vi "GEA2 Read ERD Multiple Messages.vi"(0 "GEA2 Reference In":refnum<k24>, 1 "Retry Count":i32=2 min=0 max=255 step=1, 2 "Read Timeout (ms)":u32=500, 5 "GEA Inputs":T4 {"Destination" format="%.0x"; "Source" format="%.0x"}, 7 "Read ERD List":T2[](array[typedef]) {"ERD Number" format="%.0x"}, 11 "Error In":errorcluster, 12 "#ERDs per message":i32=1 min=1 step=1, 13 "Verify ERD Response?":bool=TRUE, 14 "Low Level Retry Count":u8=3 min=1 step=1) -> (4 "GEA2 Reference Out":refnum<k24>, 6 "Raw Data Out":string[](array[string]), 8 "ERD Data Out":T1[](array[typedef]) {"ERD Number" format="%.0x"}, 15 "Error Out":errorcluster)   [LabVIEW 2016, in "GEA2_Toolkit.lvlib"]
uses:
  library/GEA2_Toolkit.lvlib
  C:/Users/220038920/Desktop/GEA3 Toolkit/GEA3 DLL Source/GeaCommunication.dll
  GEA3 DLL Source/GeaCommunication.dll
  type defs/Source_Destination.ctl
  type defs/ERD Read Data In.ctl
  type defs/Data Type.ctl
  type defs/ERD Read Data Out.ctl
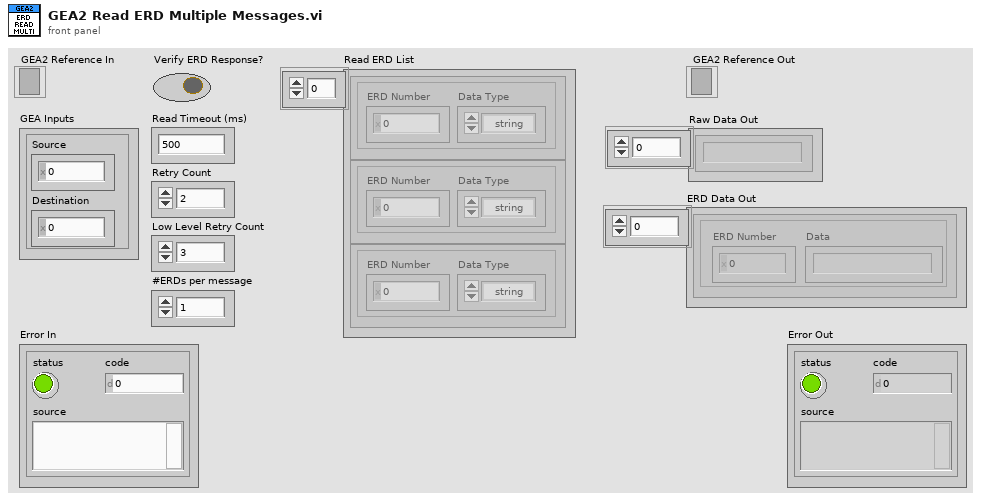
[diagram p1: front panel]
types:
  T1 = typedef "GEA2_Toolkit.lvlib/ERD Read Data Out.ctl" = cluster{"ERD Number":u16, "Data":string}
  T2 = typedef "GEA2_Toolkit.lvlib/ERD Read Data In.ctl" = cluster{"ERD Number":u16, "Data Type":T3}
  T3 = typedef "GEA2_Toolkit.lvlib/Data Type.ctl" = enum16{"string", "boolean", "uint8_t", "uint16_t", "uint32_t", "uint64_t", "int8_t", "int16_t", "int32_t", "int64_t"}
  T4 = typedef "GEA2_Toolkit.lvlib/Source_Destination.ctl" = cluster{"Source":u8, "Destination":u8}
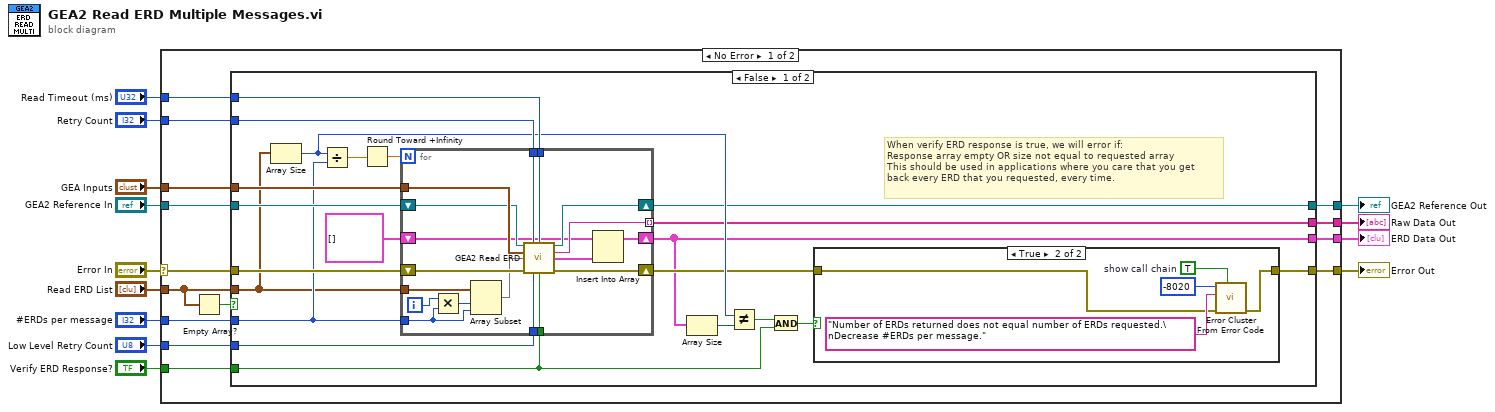
[diagram p0: block diagram]
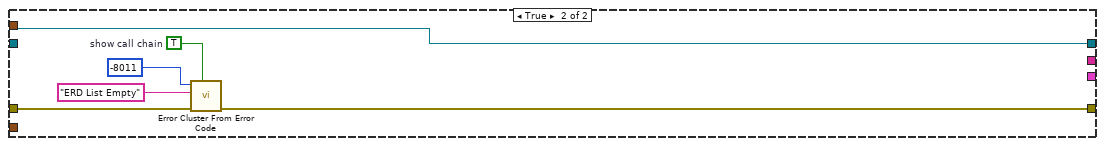
[diagram p3: hidden frame]
diagram:
  n1 = case shown="No Error" "Error In" {
    selector: "Error In" -> [w14 w79]
    tunnel: [w27 w80] -> w13
    tunnel: [w26 w79] -> w12
    tunnel: "Verify ERD Response?" -> [w25 _]
    tunnel: "GEA Inputs" -> [w24 _]
    tunnel: "Read Timeout (ms)" -> [w23 _]
    tunnel: "Retry Count" -> [w22 _]
    tunnel: "GEA2 Reference In" -> [w21 w80]
    tunnel: "#ERDs per message" -> [w20 _]
    tunnel: [w19 _] -> w5
    tunnel: [w18 _] -> w4
    tunnel: "Read ERD List" -> [w17 _]
    tunnel: "Low Level Retry Count" -> [w15 _]
    frame No Error {
      n2 = Empty Array?(array=w17) -> (empty?=w16:bool)
      n3 = case shown="False" w16 {
        tunnel: [w31 w73] -> w27
        tunnel: w14 -> [w48 w75]
        tunnel: [w34 w74] -> w26
        tunnel: w25 -> [w30 _]
        tunnel: w24 -> [w47 _]
        tunnel: w23 -> [w46 _]
        tunnel: w22 -> [w45 _]
        tunnel: w21 -> [w44 w73]
        tunnel: w20 -> [w41 _]
        tunnel: [w32 _] -> w19
        tunnel: [w33 _] -> w18
        tunnel: w17 -> [w38 _]
        tunnel: w15 -> [w39 _]
        frame False {
          # "When verify ERD response is true, we will error if:\nResponse array empty OR size not equal to requested array\nThis should be used in applications where you care that you get\nback every ERD that you requested, every time."
          n4 = Array Size(array=w38) -> (size(s)=w37:i32)
          n5 = Divide(x=w37, y=w41) -> (x/y=w43:dbl)
          n6 = Round Toward +Infinity(x=w43) -> (ceil(x): smallest int >= x=w42:dbl)
          n7 = for {
            N: w42 -> [_]
            tunnel: w30 -> [w69]
            tunnel: w47 -> [w68]
            tunnel: [w67] -> w32 mode=indexing
            tunnel: w46 -> [w66]
            tunnel: w45 -> [w65]
            shift-right: [w72] -> w31
            shift-left: w44 -> [w60]
            shift-right: [w70] -> w35
            shift-left: w48 -> [w71]
            tunnel: w38 -> [w64]
            tunnel: w41 -> [w63]
            shift-right: [w56] -> w33
            shift-left: T1[] [] -> [w58]
            tunnel: w39 -> [w55]
            i -> [w62]
            n8 = Multiply(x=w62, y=w63) -> (x*y=w61:i32)
            n9 = Array Subset(array=w64, index=w61, length=w63) -> (w59:T2[])
            n10 = call "GEA2 Read ERD.vi"("GEA2 Reference In"=w60, "Retry Count"=w65, "Read Timeout (ms)"=w66, "GEA Inputs"=w68, "Read ERD List"=w59, "Error In"=w71, "Low Level Tries"=w55, "Verify ERD Response?"=w69) -> ("GEA2 Reference Out"=w72:refnum<k24>, "Raw Data Out"=w67:string, "ERD Data Out"=w57:T1[], "Error Out"=w70:errorcluster)  [unwired: 4 in]
            n11 = Insert Into Array(array=w58, new element=w57) -> (w56:T1[])  [unwired: 1 in]
          }
          n12 = Array Size(array=w33) -> (size(s)=w36:i32)
          n13 = Not Equal?(x=w37, y=w36) -> (x != y?=w28:bool)
          n14 = And(x=w28, y=w30) -> (x .and. y?=w29:bool)
          n15 = case shown="True" w29 {
            tunnel: w35 -> [w49 w51]
            tunnel: [w49 w50] -> w34
            frame False {
            }
            frame True {
              w54 = TRUE  # show call chain
              n16 = call <vilib>:"Error Cluster From Error Code.vi"("show call chain? (False)"=w54, "error in (no error)"=w51, "error message (\"\")"="Number of ERDs returned does not equal number of ERDs requested.\nDecrease #ERDs per message." ("error message (\"\")"), "error code (0)"=-8020) -> ("error out"=w50:errorcluster)  [unwired: 5 in]
            }
          }
        }
        frame True {
          w76 = TRUE  # show call chain
          n17 = call <vilib>:"Error Cluster From Error Code.vi"("show call chain? (False)"=w76, "error in (no error)"=w75, "error message (\"\")"="ERD List Empty" ("error message (\"\")"), "error code (0)"=-8011) -> ("error out"=w74:errorcluster)  [unwired: 5 in]
        }
      }
    }
    frame Error {
    }
  }
  "GEA2 Reference Out" <- w13
  "Error Out" <- w12
  "Raw Data Out" <- w5
  "ERD Data Out" <- w4
